vi "ParseStates.vi"(0 "base path":path) -> (1 "CA STATES":string[][](array[string]), 2 "CA PROCESSES":string[](array[string])=["Èíèöèàëèçàöèÿ", "ÎñòàíîâÂñåõÏðîöåññîâÈñòàðòÏðîöÈíèöèàëèçàöèÿ", "ÊîíòðîëüÄîñòîâåðíîñòè", "ÊîíòðîëüÄîñòîâåðíîñòèÎòêðûòèÿÇàòâîðàÂàêóóìíîãî", "ÊîíòðîëüÄîñòîâåðíîñòèÎòêðÇàòÂàêóóìíîãî", "ÊîíòðîëüÄîñòîâåðíîñòèÇàêðÇàòÂàêóóìíîãî", "ÊîíòðîëüÄîñòîâåðíîñòèÑîñòîÿíèÿÑàïóíà", "ÊîíòðîëüÄîñòîâåðíîñòèÑîñòîÿíèÿÓñòðîéñòâàÏëàâÏóñêà", "ÊîíòðîëüÄîñòîâåðíîñòèÑîñòîÿíèÿÏèòàíèÿÂàêóóìíîãîÍàñîñà", "ÊîíòðîëüÄîñòîâåðíîñòèÑîñòîÿíèÿÏèòàíèÿÂåíòèëÿòîðà", "ÊîíòðîëüÄîñòîâåðíîñòèÑîñòîÿíèÿÏèòàíèÿÐåãÒåìïåðàòóðû", "ÊîíòðîëüÄîñòîâåðíîñòèÑîñòîÿíèÿÏèòàíèÿÐåãÓðîâíÿ", "ÊîíòðîëüÄîñòîâåðíîñòèÓðîâíÿÂîäûÌèíèìóì", "ÊîíòðîëüÄîñòîâåðíîñòèÓðîâíÿÂîäûÌàêñèìóì", "ÊîíòðîëüÄîñòîâåðíîñòèÑîñòîÿíèÿÏèòàíèÿÍàñÎõëàæäåíèÿ", "×òåíèåÔàêòÏàðàìåòðîâ_ñ_Äàò÷èêîâ", "ÐÅÃÓËßÒÎÐ_ÒÐÀÔÈÊÀ", "×òåíèåÊîëüöåâîãîÁóôåðà", "ÎáðàáîòêàÊîìàíäÈçìåíåíèÿÍÏ_îò_ÃÓÈ", "ÎáðàáîòêàÊîìàíäÓïðàâëåíèÿ_îò_ÃÓÈ", "ÊîíòðîëüÈçìåíåíèÿ_ÔÏ_P_ÂáàêåÊîìïðåññîðà", "ÊîíòðîëüÈçìåíåíèÿ_ÔÏ_P_Âïàòðóáêå", "ÊîíòðîëüÈçìåíåíèÿ_ÔÏ_T_Âðóáàøêå", "ÊîíòðîëüÈçìåíåíèÿ_ÔÏ_T_Âáàêå", "ÊîíòðîëüÈçìåíåíèÿ_ÔÏ_P_ÂòðóáåÑèäåð", "ÊîíòðîëüÂåëè÷èíûÎòêà÷êèÂàóóìíîéÒðóáûÑèäåðîñòàòà", "ÊîíòðîëüÃîòîâíîñòèÂàêóóìà_â_Âàêóóìíîé_Òðóáå", "ÊîíòðîëüÓðîâíÿÂîäûÁàêàÎõëàæäåíèÿ", "ÊîíòðîëüÒåìïåðàòóðûÂîäûÁàêàÎõëàæäåíèÿ", "ÊîíòðîëüÒåìïåðàòóðûÐóáàøêèÎõëàæäåíèÿ", "ÊîíòðîëüÄàâëåíèÿÂáàêåÊîìïðåññîðà", "ÂÊË_ÏÈÒ_ÂÅÍÒÈËßÒÎÐ", "ÂÛÊ_ÏÈÒ_ÂÅÍÒÈËßÒÎÐ", "ÊîíòðîëüÑîñòîÿíèÿÏèòàíèÿÂåíòèëÿòîðà", "ÊîíòðîëüÑïîíòàííîãîÂûêëþ÷åíèÿÂåíòèëÿòîðà", "ÊîíòðîëüÑïîíòàííîãîÂêëþ÷åíèÿÂåíòèëÿòîðà", "ÊîíòðîëüÑîñòîÿíèÿÇàòâîðàÂàêóóìíîãî", "ÎÒÊÐ_ÇÀÒÂÎÐ_ÂÀÊ", "ÇÀÊÐ_ÇÀÒÂÎÐ_ÂÀÊ", "ÊîíòðîëüÑïîíòàííîãîÇàêðûòèÿÇàòâîðàÂàêóóìíîãî", "ÊîíòðîëüÑïîíòàííîãîÎòêðûòèÿÇàòâîðàÂàêóóìíîãî", "ÎÒÊÐ_ÑÀÏÓÍ", "ÇÀÊÐ_ÑÀÏÓÍ", "ÊîíòðîëüÑîñòîÿíèÿÏèòàíèÿÑàïóíà", "ÊîíòðîëüÑïîíòàííîãîÇàêðûòèÿÑàïóíà", "ÊîíòðîëüÑïîíòàííîãîÎòêðûòèÿÑàïóíà", "ÂÊË_ÏÈÒ_ÂÀÊ_ÍÀÑÎÑÀ", "ÂÛÊ_ÏÈÒ_ÂÀÊ_ÍÀÑÎÑÀ", "ÊîíòðîëüÑîñòîÿíèÿÏèòàíèÿÂàêóóìíîãîÍàñîñà", "ÊîíòðîëüÑïîíòàííîãîÂûêëþ÷åíèÿÂàêÍàñîñà", "ÊîíòðîëüÑïîíòàííîãîÂêëþ÷åíèÿÂàêÍàñîñà", "ÂÊË_ÏÈÒ_ÐÅÃ_Ò", "ÂÛÊ_ÏÈÒ_ÐÅÃ_Ò", "ÊîíòðîëüÑîñòîÿíèÿÏèòàíèÿÐÅÃ_Ò", "ÊîíòðîëüÑïîíòàííîãîÂûêëþ÷åíèÿÐÅÃ_Ò", "ÊîíòðîëüÑïîíòàííîãîÂêëþ÷åíèÿÐÅÃ_Ò", "ÂÊË_ÏÈÒ_ÐÅÃ_ÓÐ", "ÂÛÊ_ÏÈÒ_ÐÅÃ_ÓÐ", "ÊîíòðîëüÑîñòîÿíèÿÏèòàíèÿÐÅÃ_ÓÐ", "ÊîíòðîëüÑïîíòàííîãîÂûêëþ÷åíèÿÐÅÃ_ÓÐ", "ÊîíòðîëüÑïîíòàííîãîÂêëþ÷åíèÿÐÅÃ_ÓÐ", "ÂÊË_ÏÈÒ_ÍÀÑ_ÎÕË", "ÂÛÊ_ÏÈÒ_ÍÀÑ_ÎÕË", "ÊîíòðîëüÑîñòîÿíèÿÏèòàíèÿÍÀÑ_ÎÕË", "ÊîíòðîëüÑïîíòàííîãîÂûêëþ÷åíèÿÍàñîñàÎõëàæäåíèÿ", "ÊîíòðîëüÑïîíòàííîãîÂêëþ÷åíèÿÍàñîñàÎõëàæäåíèÿ", "ÂÊË_ÓÑÒÐ_ÏËÀÂ_ÏÓÑÊÀ", "ÂÛÊ_ÓÑÒÐ_ÏËÀÂ_ÏÓÑÊÀ", "ÊîíòðîëüÑîñòîÿíèÿÏèòàíèÿÏËÀÂ_ÏÓÑÊÀ", "ÊîíòðîëüÑïîíòàííîãîÂûêëþ÷åíèÿÏëàâíÏóñêà", "ÊîíòðîëüÑïîíòàííîãîÂêëþ÷åíèÿÏëàâíÏóñêà", "ÂÊË_ÂÀÊÓÓÌÈÐÎÂÀÍÈÅ_ÒÐÓÁÛ", "ÂÛÊ_ÂÀÊÓÓÌÈÐÎÂÀÍÈÅ_ÒÐÓÁÛ", "ÂÊË_ÂÀÊÓÓÌÍÓÞ_ÏÎÄÑÈÑÒÅÌÓ", "ÂÛÊ_ÂÀÊÓÓÌÍÓÞ_ÏÎÄÑÈÑÒÅÌÓ"])   [LabVIEW 2010]
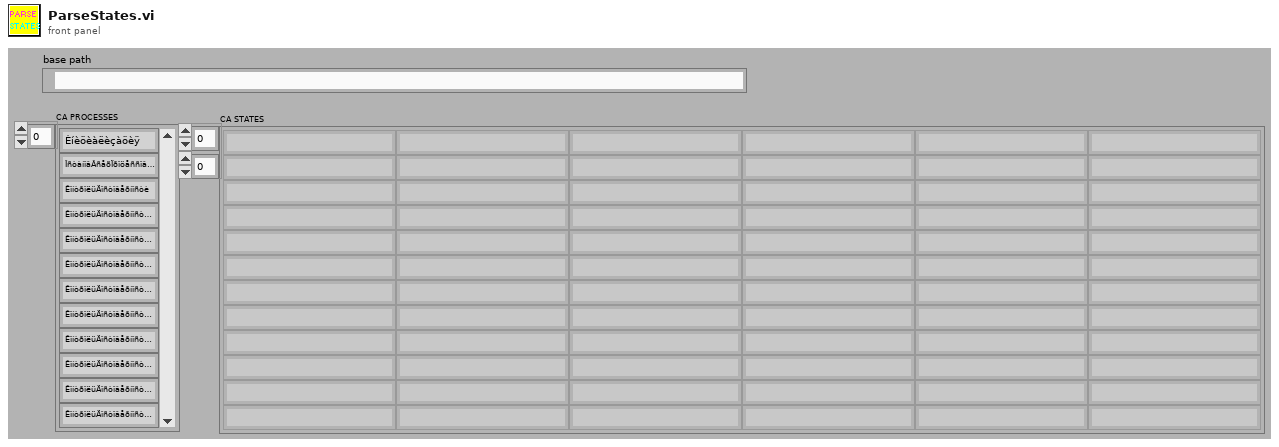
[diagram p1: front panel]
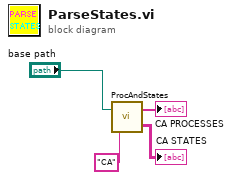
[diagram p0: block diagram]
diagram:
  n1 = call "ProcAndStates.vi"("FileName"="CA", "base path"="base path") -> ("STATES"=→"CA STATES":string[][], "PROCESSES"=→"CA PROCESSES":string[])
